vi "String to IP.vi"(11 "IP Address":string="10.155.16.12") -> (0 "IP4":i32, 1 "IP3":i32, 2 "IP2":i32, 3 "IP1":i32)   [LabVIEW 2016]
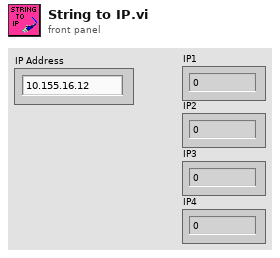
[diagram p1: front panel]
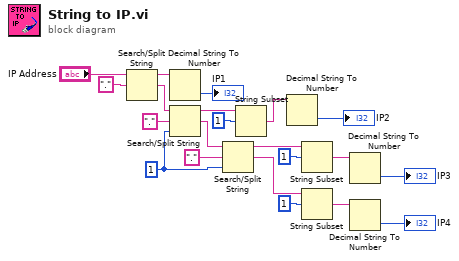
[diagram p0: block diagram]
diagram:
  w16 = 1 ("offset (0)")
  n1 = Search/Split String(string="IP Address", search string/char (-)=".") -> (substring before match=w10:string, match + rest of string=w19:string)  [unwired: 1 in, 1 out]
  n2 = Decimal String To Number(string=w10) -> (number=→"IP1":i32)  [unwired: 2 in, 1 out]
  n3 = Search/Split String(string=w19, search string/char (-)=".", offset (0)=w16) -> (substring before match=w14:string, match + rest of string=w17:string)  [unwired: 1 out]
  n4 = Search/Split String(string=w17, search string/char (-)=".", offset (0)=w16) -> (substring before match=w11:string, match + rest of string=w1:string)  [unwired: 1 out]
  n5 = String Subset(string=w14, offset (0)=1) -> (substring=w6:string)  [unwired: 1 in]
  n6 = Decimal String To Number(string=w6) -> (number=→"IP2":i32)  [unwired: 2 in, 1 out]
  n7 = String Subset(string=w11, offset (0)=1) -> (substring=w5:string)  [unwired: 1 in]
  n8 = String Subset(string=w1, offset (0)=1) -> (substring=w3:string)  [unwired: 1 in]
  n9 = Decimal String To Number(string=w5) -> (number=→"IP3":i32)  [unwired: 2 in, 1 out]
  n10 = Decimal String To Number(string=w3) -> (number=→"IP4":i32)  [unwired: 2 in, 1 out]
